vi "Depth Image Continuous Aquisition.vi"() -> ()   [LabVIEW 2011]
uses:
  <vilib>/LabVIEW Hacker/LVH-Interface-for-Kinect/LVH-Interface-for-Kinect.lvlib
  <vilib>/LabVIEW Hacker/LVH-Interface-for-Kinect/Public/lib/freenect_sync.dll
panel:
  out "Kinect Depth Image":T1(plugin-control)
  out "Frame Number":i32
  in  "Stop Button":bool
  # "This example continuously acquires the depth image from the Kinect ."
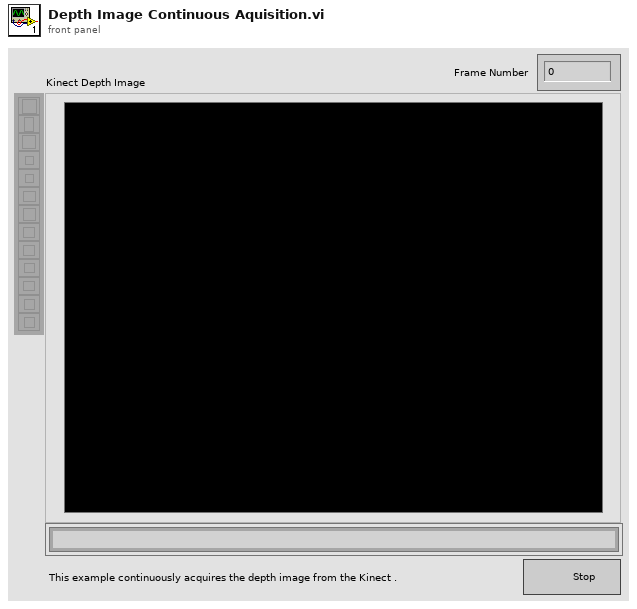
[diagram p1: front panel]
types:
  T1 = typedef "IMAQ Image.ctl" = refnum<image>
  T2 = typedef "Image Type" = u32
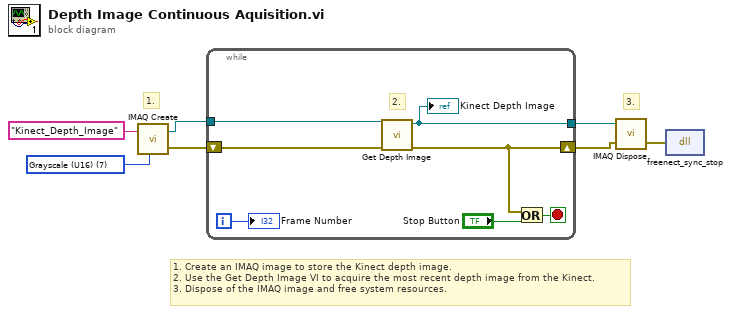
[diagram p0: block diagram]
diagram:
  w3 = T2 7 items=["Grayscale (U8)", "Grayscale (I16)", "Grayscale (SGL)", "Complex (CSG)", "RGB (U32)", "HSL (U32)", "RGB (U64)", "Grayscale (U16)"] ("Image Type")
  # "1. Create an IMAQ image to store the Kinect depth image.\n2. Use the Get Depth Image VI to acquire the most recent depth image from the Kinect.\n3. Dispose of the IMAQ image and free system resources."
  # "3."
  # "1."
  n1 = call "IMAQ Create"("Image Name"="Kinect_Depth_Image", "Image Type"=w3) -> ("New Image"=w7:T1, "error out"=w5:errorcluster)  [unwired: 3 in]
  n2 = while {
    tunnel: w7 -> [w13]
    tunnel: [w8] -> w6
    shift-right: [w10] -> w2
    shift-left: w5 -> [w9]
    i -> [w14]
    stop <- w11 stop-if-true
    # "2."
    n3 = call <vilib>:"Get Depth Image.vi"("Error In"=w9, "Image"=w13) -> ("Error Out"=w10:errorcluster, "Image Out"=w8:T1)  [unwired: 7 in, 1 out]
    "Kinect Depth Image" <- w8
    n4 = Or(x=w10, y="Stop Button") -> (x .or. y?=w11:bool)
    "Frame Number" <- w14
  }
  n5 = call "IMAQ Dispose"("Image"=w6, "error in (no error)"=w2) -> ("error out"=w1:errorcluster)  [unwired: 4 in]
  n6 = dll-call lib="C:/Program Files/National Instruments/LabVIEW 2011/vi.lib/LabVIEW Hacker/LVH-Interface-for-Kinect/Public/lib/freenect_sync.dll" fn="freenect_sync_stop"(error in=w1) -> ()  [unwired: 3 in, 2 out]
